vi "GetSetRegion.vi"(7 "Set":bool, 8 "error in (no error)":errorcluster, 9 "Image Size":T1, 10 "Image Offset":T2, 11 "Camera in":refnum<class "Camera.lvclass">) -> (0 "error out":errorcluster, 1 "Image Size":T1, 2 "Image Offset":T2, 3 "Camera":refnum<class "Camera.lvclass">)   [LabVIEW 2020, in "Camera.lvclass"]
uses:
  Camera.lvclass
  Buffer/Image Size.ctl
  Image Offset.ctl
  Camera.lvclass/Camera.ctl
  bin/gindustrialcam_32-1.dll
  Buffer/Buffer.lvclass
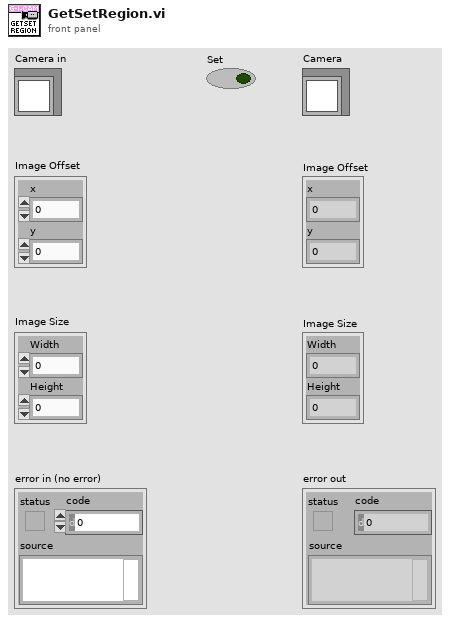
[diagram p1: front panel]
types:
  T1 = typedef "Buffer.lvclass/Image Size.ctl" = cluster{"Width":u16, "Height":u16}
  T2 = typedef "Camera.lvclass/Image Offset.ctl" = cluster{"x":i32, "y":i32}
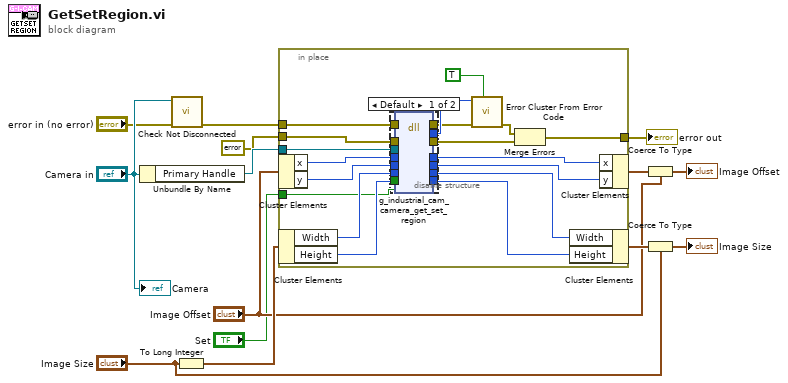
[diagram p0: block diagram]
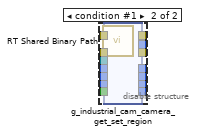
[diagram p2: hidden frame]
diagram:
  n1 = Unbundle By Name("Camera in") -> ("Primary Handle"=w10:refnum<data-value>)
  n2 = call "Check Not Disconnected.vi"("error in (no error)"="error in (no error)", "Camera in"="Camera in") -> ("error out"=w11:errorcluster)  [unwired: 9 in]
  n3 = To Long Integer(number="Image Size") -> (32bit integer=w8:cluster{"Width":i32, "Height":i32})
  n4 = in-place {
    in-place-border: [w32] -> w12
    in-place-border: w11 -> [w31]
    in-place-border: w10 -> [w30]
    in-place-border: errorcluster {"status"=FALSE, "code"=0, "source"=""} ("error constant") -> [w29]
    in-place-border: "Set" -> [w15]
    n5 = in-place-cluster #1("Image Offset") -> ("x"=w23:i32, "y"=w22:i32)
    n6 = in-place-cluster #2(w8) -> ("Width"=w21:i32, "Height"=w20:i32)
    n7 = disable-structure shown="Default" {
      disable-tunnel: w31 -> [w47 w63]
      disable-tunnel: w30 -> [w46 w62]
      disable-tunnel: w29 -> [w45 w61]
      disable-tunnel: [w44 w60] -> w27
      disable-tunnel: [w43 w59] -> w25
      disable-tunnel: [w42 w58] -> w24
      disable-tunnel: w23 -> [w41 w57]
      disable-tunnel: w22 -> [w40 w56]
      disable-tunnel: w21 -> [w39 w55]
      disable-tunnel: w20 -> [w38 w54]
      disable-tunnel: [w37 w53] -> w19
      disable-tunnel: [w36 w52] -> w18
      disable-tunnel: [w35 w51] -> w17
      disable-tunnel: [w34 w50] -> w16
      disable-tunnel: w15 -> [w33 w49]
      frame condition #0 (active) {
        n8 = dll-call lib="C:/serenial/lib/g-industrial-camera/LabVIEW/g_industrial_cam/bin/gindustrialcam_*-1.*" fn="g_industrial_cam_camera_get_set_region"(error in=w47, "err"=w45, "edvr"=w46, "x"=w41, "y"=w40, "width"=w39, "height"=w38, "set"=w33) -> (error out=w42:errorcluster, "Mg_Error"=w43:i32, "err"=w44:errorcluster, "x"=w37:i32, "y"=w36:i32, "width"=w35:i32, "height"=w34:i32)  [unwired: 4 in, 1 out]
      }
      frame condition #1 {
        n9 = call "RT Shared Binary Path.vi"() -> ("Path"=w48:path)
        n10 = dll-call lib="C:/serenial/lib/g-industrial-camera/LabVIEW/g_industrial_cam/bin/gindustrialcam_*-1.*" fn="g_industrial_cam_camera_get_set_region"(path in=w48, error in=w63, "err"=w61, "edvr"=w62, "x"=w57, "y"=w56, "width"=w55, "height"=w54, "set"=w49) -> (error out=w58:errorcluster, "Mg_Error"=w59:i32, "err"=w60:errorcluster, "x"=w53:i32, "y"=w52:i32, "width"=w51:i32, "height"=w50:i32)  [unwired: 3 in, 1 out]
      }
    }
    n11 = call <vilib>:"Error Cluster From Error Code.vi"("show call chain? (False)"=TRUE, "error in (no error)"=w24, "error code (0)"=w25) -> ("error out"=w26:errorcluster)  [unwired: 6 in]
    n12 = Merge Errors(w26, w27) -> (w32:errorcluster)
    n13 = in-place-cluster #2("Width"=w17, "Height"=w16) -> (w7:cluster{"Width":i32, "Height":i32})
    n14 = in-place-cluster #1("x"=w19, "y"=w18) -> (w5:T2)
  }
  "error out" <- w12
  n15 = Coerce To Type(0:w5, 1:"Image Offset") -> (2:→"Image Offset":T2)
  n16 = Coerce To Type(0:w7, 1:"Image Size") -> (2:→"Image Size":T1)
  "Camera" <- "Camera in"
